vi "CMD_0.vi"() -> (3 "JSON String":string)   [LabVIEW 2025]
uses:
  <vilib>/addons/_JKI.lib/Serialization/JSON/JKI JSON Serialization.lvlib
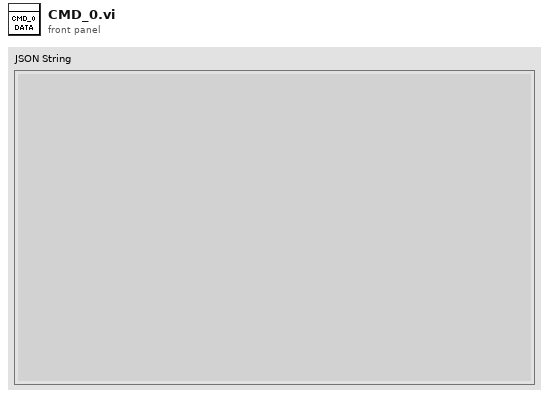
[diagram p1: front panel]
types:
  T1 = cluster{"ID":string, "TO":string, "FROM":string, "CMD":u32, "CONTENT":variant, "STATUS":string, "ERRCODE":string, "ERRMSG":string, "TIMESTAMP":u32}
  T2 = cluster{"HOSTNAME":string, "MAC":string, "IP":string}
  T3 = cluster{"HOSTNAME":string, "MAC":string, "IP":string}[]
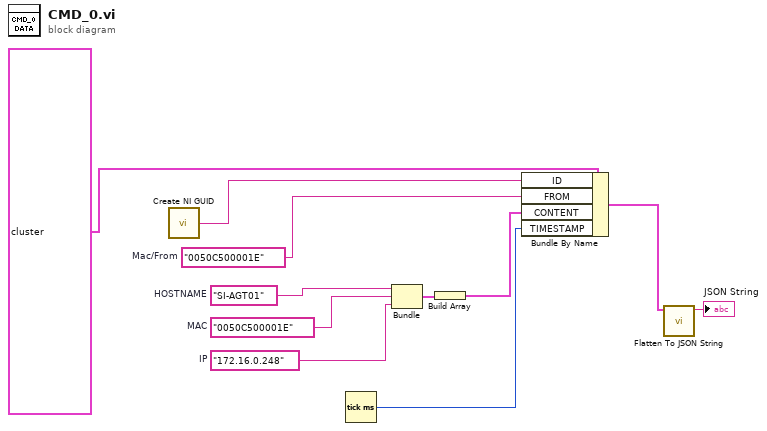
[diagram p0: block diagram]
diagram:
  w7 = "0050C500001E"  # MAC
  w8 = "SI-AGT01"  # HOSTNAME
  w6 = "172.16.0.248"  # IP
  w9 = "0050C500001E"  # Mac/From
  n1 = call <vilib>:"Create NI GUID.vi"() -> ("NI GUID"=w10:string)
  n2 = Tick Count (ms)() -> (millisecond timer value=w4:u32)
  n3 = Bundle("HOSTNAME"=w8, "MAC"=w7, "IP"=w6) -> (w2:T2)  [unwired: 1 in]
  n4 = Build Array(w2) -> (w1:T3)
  n5 = Bundle By Name(cluster=T1 {"ID"="", "TO"="", "FROM"="", "CMD"=0, "CONTENT"=variant, "STATUS"="", "ERRCODE"="", "ERRMSG"="", "TIMESTAMP"=0}, "ID"=w10, "FROM"=w9, "CONTENT"=w1, "TIMESTAMP"=w4) -> (w5:T1)
  n6 = call <vilib>:"Flatten To JSON String.vi"("Variant"=w5) -> ("JSON String"=→"JSON String":string)  [unwired: 9 in, 1 out]
